vi "USGlobalSat GPS.vi"() -> ()   [LabVIEW 2012]
uses:
  <vilib>/Platform/TimedLoop/XDataNode/timing_clust.ctl
  <vilib>/Platform/TimedLoop/XDataNode/nitl_modes.ctl
  <vilib>/Platform/TimedLoop/XDataNode/wakeup.ctl
  <vilib>/Platform/TimedLoop/XDataNode/XDataNode.xnode
  USGlobalSat.lvlib
  <vilib>/Platform/TimedLoop/XDataNode/XDNodeRunTimeDep.lvlib
panel:
  in  "stop?":bool
  in  "error in (no error)":errorcluster
  out "GPS Data":T1 {"Time"."GPS Time of Week" format="%.3f"; "Velocity, Correction & SET"."Extended Navigation Mode" items=["Non Differential"=0, "Code (RTCM Type 1 & 9)"=1, "Code, Single Frequency (WAAS)"=2, "Code, Dual Frequency (WAAS)"=3, "Code, Single Frequency (WCT)"=4, "Code/RCP, Dual Frequency (WCT)"=5, "Code, Single Frequency (RTG)"=6, "Code (RTCM Type 1 & 9) Dual Frequency"=10, "Code/RCP, Dual Frequency (RTG)"=11, "Code, Single Frequency (NCT-RTK)"=12, "Code, Single Frequency (RTCM 18 & 19)"=13, "Code, Single Frequency (RTCM 21 & 22)"=14, "Code, Single Frequency (CMR)"=15, "Code, Dual Frequency (NCT-RTK)"=16, "Code, Dual Frequency (RTCM 18 & 19)"=17, "Code, Dual Frequency (RTCM 20 & 21)"=18, "Code, Dual Frequency (CMR)"=19, "RTK (NCT-RTK)"=20, "RTK (RTCM 18 & 19)"=21, "RTK (RTCM 20 & 21)"=22, "RTK (CMR)"=23, "Code, Single Frequency with SET (RTG)"=24, "Code/RCP, Dual Frequency with SET (RTG)"=25, "RTK Extend"=26]; "Altitude" format="%#_18g"; "Longitude" format="%#_18g"; "Latitude" format="%#_18g"}
  in  "Debug":bool
  in  "VISA resource name":refnum<visa-resource-name>
  out "error out":errorcluster
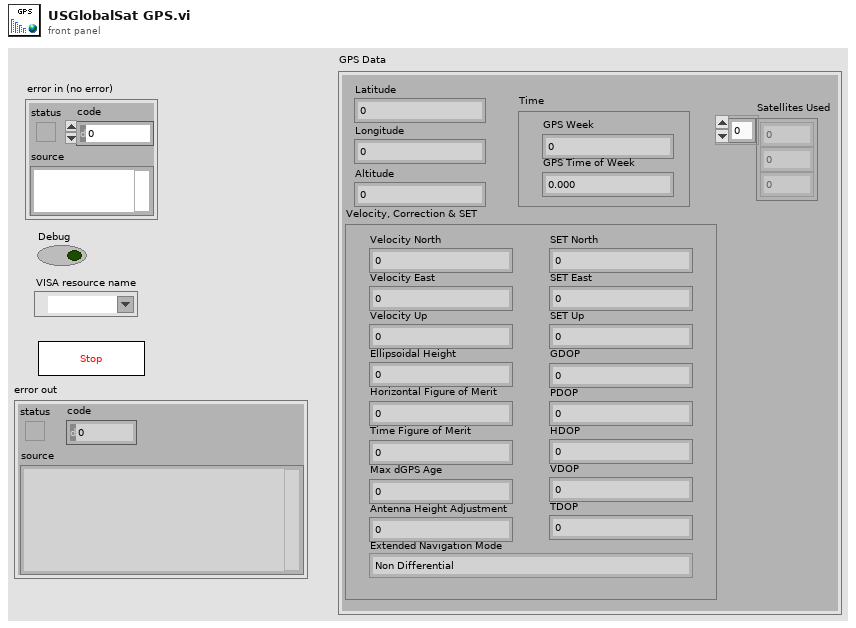
[diagram p1: front panel]
types:
  T1 = cluster{"Latitude":dbl, "Longitude":dbl, "Altitude":dbl, "Velocity, Correction & SET":cluster{"Velocity North":dbl, "Velocity East":dbl, "Velocity Up":dbl, "Ellipsoidal Height":dbl, "GDOP":sgl, "PDOP":sgl, "HDOP":sgl, "VDOP":sgl, "TDOP":sgl, "Horizontal Figure of Merit":u8, "Time Figure of Merit":u8, "Max dGPS Age":sgl, "Extended Navigation Mode":u8, "Antenna Height Adjustment ":dbl, "SET North":i32, "SET East":i32, "SET Up":i32}, "Time":cluster{"GPS Week":u16, "GPS Time of Week":sgl}, "Satellites Used":i32[]}
  T2 = typedef "XDNodeRunTimeDep.lvlib/timing_clust.ctl" = cluster{"Expected End [f-1]":u64, "Actual End [f-1]":u64, "Finished Late? [f-1]":bool, "Expected End [i-1]":u64, "Actual End [i-1]":u64, "Finished Late? [i-1]":bool, "Expected Start [i]":u64, "Actual Start [i]":u64, "Expected Start [f]":u64, "Actual Start [f]":u64, "Source Name":string, "Structure Name":string, "Period":i64, "Deadline":i64, "Offset":i64, "Start":i64, "Priority":i32, "Timeout":i32, "Mode":T3, "Wakeup Reason":T4, "Error":errorcluster, "Source Type":string, "Secondary Source Type":string, "Global End Time":u64, "Global Start Time":u64, "Frame Duration":u64, "Iteration Duration":u64, "Assigned CPU":i32, "I/O Scan Engine Mode":u32}
  T3 = typedef "XDNodeRunTimeDep.lvlib/nitl_modes.ctl" = enum32{"No Change", "Process missed periods, maintain original phase", "Discard missed periods, maintain original phase", "Process missed periods, ignore original phase", "Discard missed periods, ignore original phase"}
  T4 = typedef "XDNodeRunTimeDep.lvlib/wakeup.ctl" = enum32{"Normal", "Aborted", "Asynchronous wakeup", "Timing source error", "Timed loop error", "Timeout"}
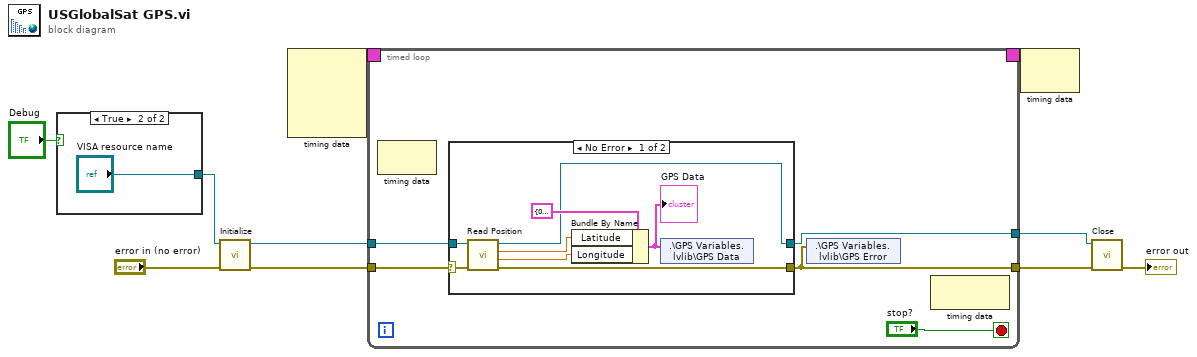
[diagram p0: block diagram]
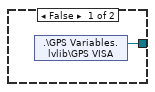
[diagram p3: hidden frame]
diagram:
  n1 = case shown="True" "Debug" {
    tunnel: [w11 "VISA resource name"] -> w9
    frame False {
      n2 = shared-variable ".\\GPS Variables.lvlib\\GPS VISA"() -> (w11:refnum<visa-resource-name>)  [unwired: 1 in, 1 out]
    }
    frame True {
    }
  }
  n3 = call "Initialize.vi"("error in (no error)"="error in (no error)", "VISA resource name"=w9) -> ("error out"=w7:errorcluster, "reference out"=w3:refnum<visa-resource-name>)  [unwired: 8 in]
  n4 = node-c288() -> (w2:T2)  [unwired: 4 in]
  n5 = timed-loop {
    tunnel: [w17] -> w5
    tunnel: w7 -> [w16]
    tunnel: [w15] -> w6
    tunnel: w3 -> [w14]
    timing: w2 -> [_]
    timing-out: [_] -> w1
    stop <- "stop?" stop-if-true
    n6 = node-c288() -> ()  [unwired: 1 in, 1 out]
    n7 = case shown="No Error" w16 {
      selector: w16 -> [w27 w29]
      tunnel: [w26 w29] -> w17
      tunnel: [w21 w28] -> w15
      tunnel: w14 -> [w20 w28]
      frame No Error {
        n8 = call "Read Position.vi"("error in (no error)"=w27, "VISA resource name"=w20) -> ("error out"=w26:errorcluster, "Longitude (ddmm.mmmm)"=w23:dbl, "Lattitude (ddmm.mmmm)"=w22:dbl, "VISA resource name out"=w21:refnum<visa-resource-name>)  [unwired: 3 in, 3 out]
        n9 = Bundle By Name(cluster=T1 {"Latitude"=0.0, "Longitude"=0.0, "Altitude"=0.0, "Velocity, Correction & SET"={"Velocity North"=0.0, "Velocity East"=0.0, "Velocity Up"=0.0, "Ellipsoidal Height"=0.0, "GDOP"=0.0, "PDOP"=0.0, "HDOP"=0.0, "VDOP"=0.0, "TDOP"=0.0, "Horizontal Figure of Merit"=0, "Time Figure of Merit"=0, "Max dGPS Age"=0.0, "Extended Navigation Mode"=0, "Antenna Height Adjustment "=0.0, "SET North"=0, "SET East"=0, "SET Up"=0}, "Time"={"GPS Week"=0, "GPS Time of Week"=0.0}, "Satellites Used"=[]} ("GPS Data Cluster"), "Latitude"=w22, "Longitude"=w23) -> (w25:T1)
        "GPS Data" <- w25
        n10 = shared-variable ".\\GPS Variables.lvlib\\GPS Data"(w25) -> ()  [unwired: 1 in, 1 out]
      }
      frame Error {
      }
    }
    n11 = shared-variable ".\\GPS Variables.lvlib\\GPS Error"(w17) -> ()  [unwired: 1 in, 1 out]
    n12 = node-c288() -> ()  [unwired: 1 in, 1 out]
  }
  n13 = node-c288(w1) -> ()  [unwired: 1 out]
  n14 = call "Close.vi"("error in (no error)"=w5, "VISA resource name"=w6) -> ("error out"=→"error out":errorcluster)  [unwired: 9 in]
